vi "FdxCmdRxUDPGetStatusCvi.vi"(8 "error in":errorcluster, 10 "UdpHandle":u32, 11 "InstrumentHandle_port":u32) -> (0 "error out":errorcluster, 1 "MsgCount":u32, 2 "UdpHandle Out":u32, 3 "InstrumentHandle_port":u32, 4 "MsgErrorCount":u32)   [LabVIEW 2020, in "AIM664LV.lvlib"]
doc: "This function reads the status of a UDP connection oriented port."
uses:
  AIM664LV.lvlib
  AFDX_LibraryAdmin/FdxGlobalDllPath.vi
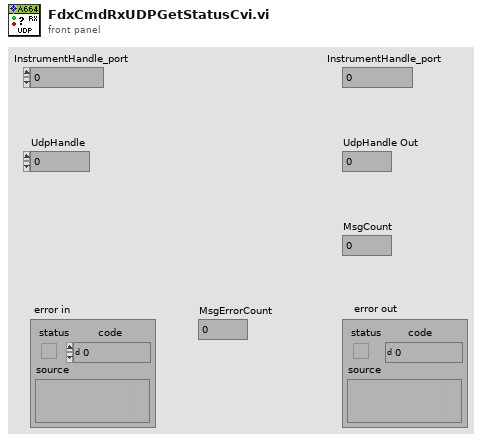
[diagram p1: front panel]
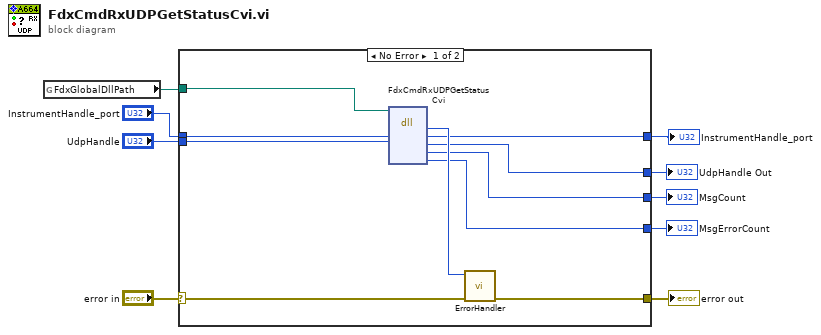
[diagram p0: block diagram]
diagram:
  n1 = global read "FdxGlobalDllPath.vi" "FdxGlobalDllPath"() -> (w7:path)
  n2 = case shown="No Error" "error in" {
    selector: "error in" -> [w18 w22]
    tunnel: [w19 w22] -> w9
    tunnel: w7 -> [w16 _]
    tunnel: "InstrumentHandle_port" -> [w15 w21]
    tunnel: [w13 w21] -> w5
    tunnel: "UdpHandle" -> [w14 w20]
    tunnel: [w12 w20] -> w3
    tunnel: [w11 _] -> w2
    tunnel: [w10 _] -> w1
    frame No Error {
      n3 = dll-call lib="aim_fdx.19.dll" fn="FdxCmdRxUDPGetStatusCvi"(path in=w16, "InstrumentHandle"=w15, "UdpHandle"=w14) -> ("status"=w17:i32, "InstrumentHandle"=w13:u32, "UdpHandle"=w12:u32, "MsgCount"=w10:u32, "MsgErrorCount"=w11:u32)  [unwired: 4 in, 2 out]
      n4 = call "ErrorHandler.vi"("error in"=w18, "AIM Error"=w17) -> ("error out"=w19:errorcluster)  [unwired: 9 in]
    }
    frame Error {
    }
  }
  "error out" <- w9
  "InstrumentHandle_port" <- w5
  "UdpHandle Out" <- w3
  "MsgCount" <- w1
  "MsgErrorCount" <- w2
